vi "ContextHelp_SplitString.vi"(0 "string":string, 1 "Max string length":i32=40) -> (14 "Array":string[](array[string]))   [LabVIEW 2014]
panel:
  out "Array 2":i32[](array[numeric])
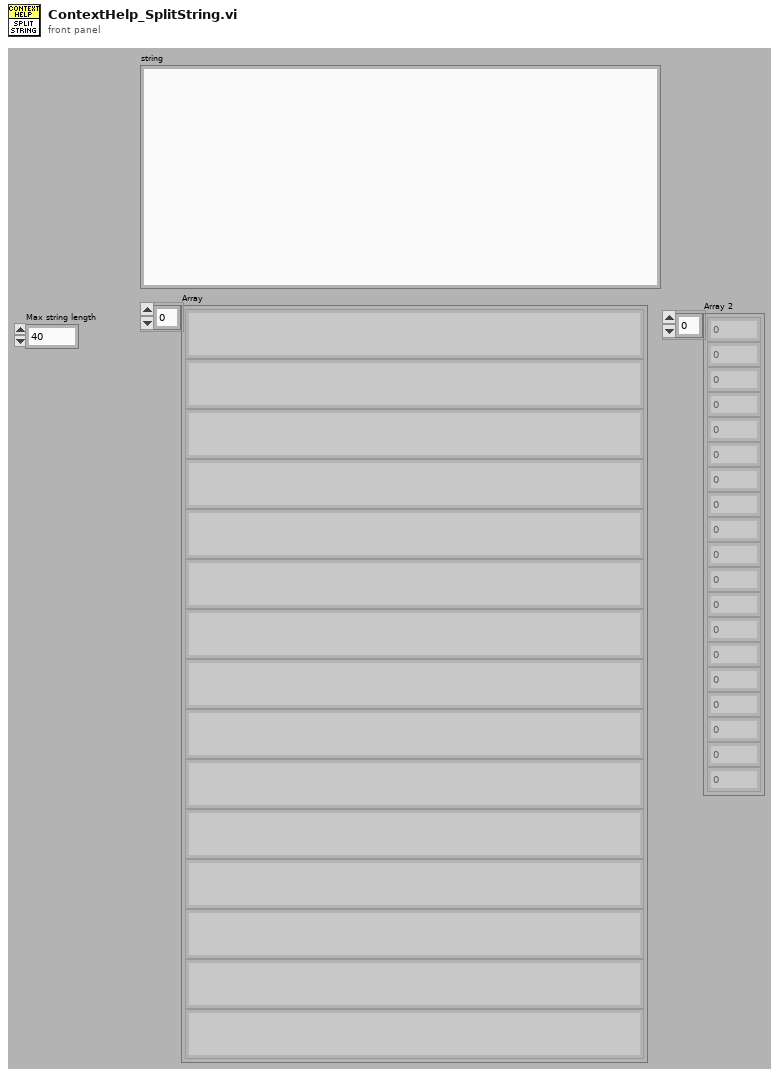
[diagram p1: front panel]
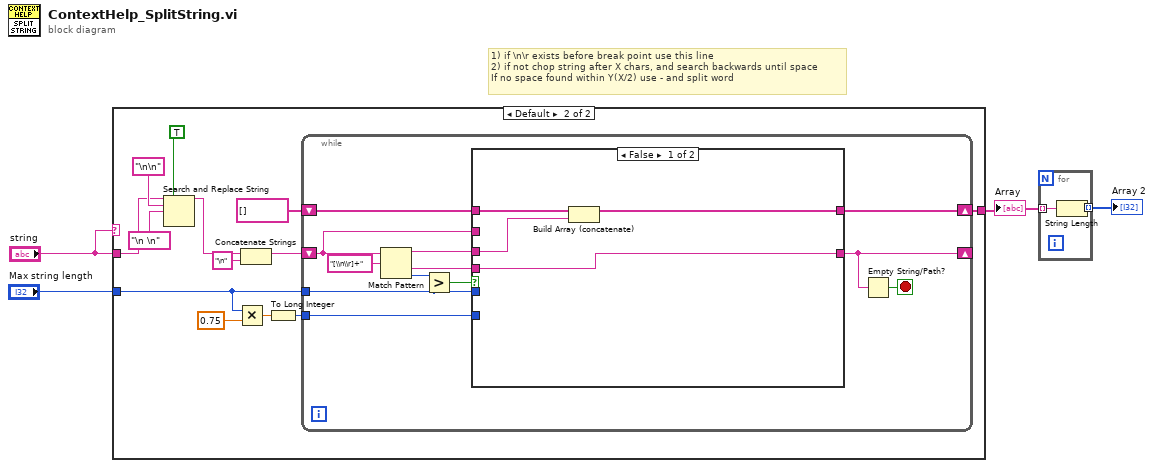
[diagram p0: block diagram]
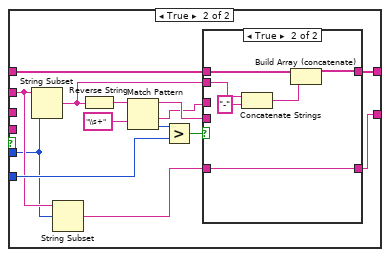
[diagram p3: hidden frame]
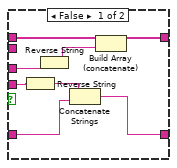
[diagram p4: hidden frame]
diagram:
  # "1) if \\n\\r exists before break point use this line\n2) if not chop string after X chars, and search backwards until space\nIf no space found within Y(X/2) use - and split word"
  n1 = case shown="Default" "string" {
    tunnel: "Max string length" -> [_ w16]
    tunnel: [_ w12] -> w3
    tunnel: "string" -> [_ w6]
    frame "" {
    }
    frame Default {
      n2 = Search and Replace String(replace all?=TRUE ("replace all? (F)"), input string=w6, search string="\n\n" ("string"), replace string="\n \n" ("string")) -> (result string=w5:string)  [unwired: 1 in, 6 out]
      n3 = Multiply(x=w16, y=0.75) -> (x*y=w14:dbl)
      n4 = Concatenate Strings(w5, "\n" ("string")) -> (w10:string)
      n5 = To Long Integer(number=w14) -> (32bit integer=w13:i32)
      n6 = while {
        shift-right: [w19] -> _
        shift-left: w10 -> [w22]
        shift-right: [w24] -> w12
        shift-left: string[] [] -> [w27]
        tunnel: w16 -> [w21]
        tunnel: w13 -> [w20]
        stop <- w18 stop-if-true
        n7 = Match Pattern(string=w22, regular expression="[\\n\\r]+") -> (before substring=w25:string, after substring=w23:string, offset past match=w28:i32)  [unwired: 2 out]
        n8 = Greater?(x=w28, y=w21) -> (0:w26:bool)
        n9 = case shown="False" w26 {
          tunnel: w27 -> [w33 w38]
          tunnel: w25 -> [w32 _]
          tunnel: [w31 w37] -> w24
          tunnel: w23 -> [w30 _]
          tunnel: [w30 w39] -> w19
          tunnel: w22 -> [_ w42]
          tunnel: w21 -> [_ w41]
          tunnel: w20 -> [_ w44]
          frame False {
            n10 = Build Array (concatenate)(w33, w32) -> (w31:string[])
          }
          frame True {
            n11 = String Subset(string=w42, length (rest)=w41) -> (substring=w34:string)  [unwired: 1 out]
            n12 = String Subset(string=w42, offset (0)=w41) -> (substring=w40:string)  [unwired: 1 out]
            n13 = Reverse String(1:w34) -> (0:w47:string)
            n14 = Match Pattern(string=w47, regular expression="\\s+") -> (before substring=w36:string, after substring=w35:string, offset past match=w45:i32)  [unwired: 2 out]
            n15 = Greater?(x=w45, y=w44) -> (0:w43:bool)
            n16 = case shown="True" w43 {
              tunnel: w40 -> [w49 w61]
              tunnel: [w48 w61] -> w39
              tunnel: w38 -> [w55 w58]
              tunnel: [w54 w57] -> w37
              tunnel: w35 -> [w53 _]
              tunnel: w36 -> [w51 _]
              tunnel: w34 -> [_ w60]
              frame False {
                n17 = Reverse String(1:w51) -> (0:w50:string)
                n18 = Reverse String(1:w53) -> (0:w52:string)
                n19 = Concatenate Strings(w50, w49) -> (w48:string)
                n20 = Build Array (concatenate)(w55, w52) -> (w54:string[])
              }
              frame True {
                n21 = Concatenate Strings(w60, "-" ("string")) -> (w56:string)
                n22 = Build Array (concatenate)(w58, w56) -> (w57:string[])
              }
            }
          }
        }
        n23 = Empty String/Path?(string/path=w19) -> (empty?=w18:bool)
      }
    }
  }
  "Array" <- w3
  n24 = for {
    tunnel: w3 -> [w63] mode=indexing
    tunnel: [w62] -> w2 mode=indexing
    n25 = String Length(string=w63) -> (length=w62:i32)
  }
  "Array 2" <- w2
